vi "SubGenerateListToOrder.vi"(8 "error in (no error)":errorcluster, 11 "SolutionBuilder in":refnum<class "SolutionBuilder.lvclass">) -> (0 "error out":errorcluster, 1 "Ordering map":T1, 3 "SolutionBuilder out":refnum<class "SolutionBuilder.lvclass">)   [LabVIEW 2019, in "SolutionBuilder.lvlib" / "SolutionBuilder.lvclass"]
uses:
  SolutionBuilder.lvclass
  OrderingMap.ctl
  ProjectItem/ProjectItem.lvclass
  ProjectItem/ProjectItem.lvclass/ProjectItem.ctl
  <vilib>/Utility/miscctls.llb/LVMapReplaceAction.ctl
  be8949a1-daf6-466d-868e-55db06778a0f.vi
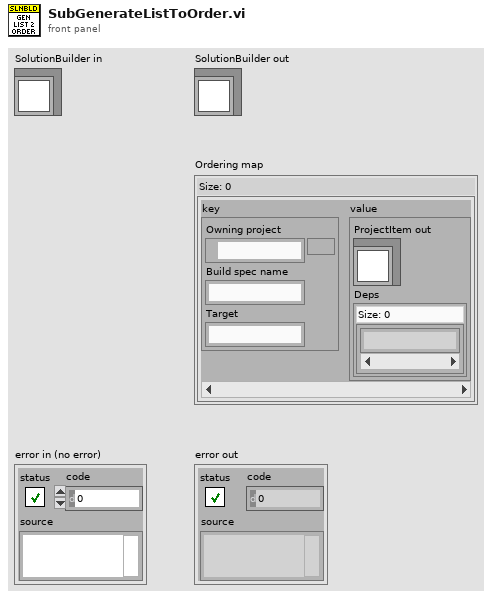
[diagram p1: front panel]
types:
  T1 = typedef "SolutionBuilder.lvlib/SolutionBuilder.lvclass/OrderingMap.ctl" = map{cluster{"Owning project":path, "Build spec name":string, "Target":string}, cluster{"ProjectItem out":refnum<class "ProjectItem.lvclass">, "Deps":set{string}}}
  T2 = typedef "SolutionBuilder.lvlib/SolutionBuilder.lvclass/ProjectItemMap.ctl" = map{path, refnum<class "ProjectItem.lvclass">[]}
  T3 = typedef "LVMapReplaceAction.ctl" = enum32{"Modify Entry only if found", "Add or Modify Entry", "Delete Entry"}
  T4 = cluster{"Owning project":path, "Build spec name":string, "Target":string}
  T5 = cluster{"ProjectItem out":refnum<class "ProjectItem.lvclass">, "Deps":set{string}}
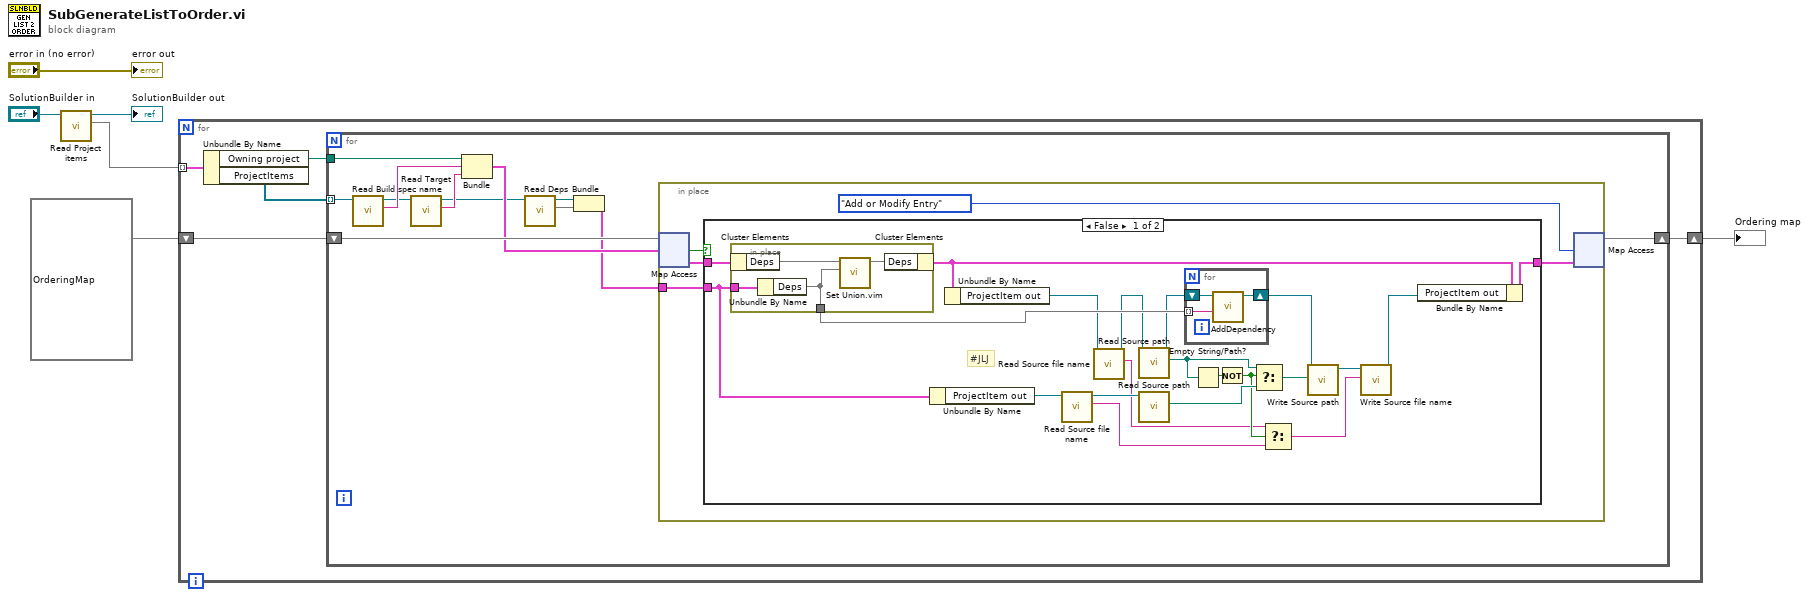
[diagram p0: block diagram]
diagram:
  n1 = call "Read Project items.vi"("SolutionBuilder in"="SolutionBuilder in") -> ("Project items"=w1:T2, "SolutionBuilder out"=→"SolutionBuilder out":refnum<class "SolutionBuilder.lvclass">)  [unwired: 9 in]
  n2 = for {
    tunnel: w1 -> [w11] mode=indexing
    shift-right: [w7] -> w4
    shift-left: T1 {} ("Ordering map") -> [w8]
    n3 = Unbundle By Name(w11) -> ("Owning project"=w10:path, "ProjectItems"=w9:refnum<class "ProjectItem.lvclass">[])
    n4 = for {
      tunnel: w9 -> [w23] mode=indexing
      tunnel: w10 -> [w19]
      shift-right: [w15] -> w7
      shift-left: w8 -> [w18]
      n5 = call "Read Build spec name.vi"("ProjectItem in"=w23) -> ("Build spec name"=w22:string, "ProjectItem out"=w14:refnum<class "ProjectItem.lvclass">)  [unwired: 9 in]
      n6 = call "Read Target.vi"("ProjectItem in"=w14) -> ("Target"=w13:string, "ProjectItem out"=w12:refnum<class "ProjectItem.lvclass">)  [unwired: 9 in]
      n7 = Bundle("Owning project"=w19, "Build spec name"=w22, "Target"=w13) -> (w17:T4)  [unwired: 1 in]
      n8 = call "Read Deps.vi"("ProjectItem in"=w12) -> ("Deps"=w20:set{string}, "ProjectItem out"=w21:refnum<class "ProjectItem.lvclass">)  [unwired: 9 in]
      n9 = Bundle("ProjectItem out"=w21, "Deps"=w20) -> (w16:T5)  [unwired: 1 in]
      n10 = in-place {
        in-place-border: w16 -> [w27]
        n11 = in-place-map #1(w18, w17) -> (w24:T5, w28:bool)  [unwired: 1 in]
        n12 = case shown="False" w28 {
          tunnel: w27 -> [w44 w57]
          tunnel: [w46 w57] -> w26
          tunnel: w24 -> [w49 _]
          frame False {
            # "#JLJ"
            n13 = in-place {
              in-place-border: w44 -> [w56]
              in-place-border: [w53] -> w48
              n14 = in-place-cluster #2(w49) -> ("Deps"=w55:set{string})
              n15 = Unbundle By Name(w56) -> ("Deps"=w53:set{string})
              n16 = call "Set Union.vim"("set 2"=w53, "set 1"=w55) -> ("union"=w54:set{string})  [unwired: 9 in]
              n17 = in-place-cluster #2("Deps"=w54) -> (w47:T5)
            }
            n18 = Unbundle By Name(w44) -> ("ProjectItem out"=w36:refnum<class "ProjectItem.lvclass">)
            n19 = Unbundle By Name(w47) -> ("ProjectItem out"=w38:refnum<class "ProjectItem.lvclass">)
            n20 = call "Read Source file name.vi"("ProjectItem in"=w36) -> ("Source file name"=w32:string, "ProjectItem out"=w35:refnum<class "ProjectItem.lvclass">)  [unwired: 9 in]
            n21 = call "Read Source file name.vi"("ProjectItem in"=w38) -> ("Source file name"=w33:string, "ProjectItem out"=w37:refnum<class "ProjectItem.lvclass">)  [unwired: 9 in]
            n22 = call "Read Source path.vi"("ProjectItem in"=w37) -> ("Source path"=w42:path, "ProjectItem out"=w45:refnum<class "ProjectItem.lvclass">)  [unwired: 9 in]
            n23 = call "Read Source path.vi"("ProjectItem in"=w35) -> ("Source path"=w41:path)  [unwired: 9 in, 1 out]
            n24 = for {
              tunnel: w48 -> [w51] mode=indexing
              shift-right: [w50] -> w39
              shift-left: w45 -> [w52]
              n25 = call "AddDependency.vi"("Dependency"=w51, "ProjectItem in"=w52) -> ("ProjectItem out"=w50:refnum<class "ProjectItem.lvclass">)  [unwired: 8 in, 1 out]
            }
            n26 = Empty String/Path?(string/path=w42) -> (empty?=w43:bool)
            n27 = Not(x=w43) -> (.not. x?=w34:bool)
            n28 = Select(t=w42, s=w34, f=w41) -> (s? t:f=w40:path)
            n29 = Select(t=w33, s=w34, f=w32) -> (s? t:f=w31:string)
            n30 = call "Write Source path.vi"("Source path"=w40, "ProjectItem in"=w39) -> ("ProjectItem out"=w30:refnum<class "ProjectItem.lvclass">)  [unwired: 9 in]
            n31 = call "Write Source file name.vi"("Source file name"=w31, "ProjectItem in"=w30) -> ("ProjectItem out"=w29:refnum<class "ProjectItem.lvclass">)  [unwired: 9 in]
            n32 = Bundle By Name(cluster=w47, "ProjectItem out"=w29) -> (w46:T5)
          }
          frame True {
          }
        }
        n33 = in-place-map #1(w26, LVMapReplaceAction."Add or Modify Entry" ("action")) -> (w15:T1)  [unwired: 2 out]
      }
    }
  }
  "Ordering map" <- w4
  "error out" <- "error in (no error)"
